vi "eventstructure.vi"() -> ()   [LabVIEW 2017]
uses:
  <vilib>/event_ctls.llb/eventsource.ctl
  <vilib>/event_ctls.llb/lveventtype.ctl
panel:
  out "Time":u32
  out "Type":T1=enum."Value Change"
  out "Source":T2 items=["LabVIEW UI"=0, "ActiveX"=1, "User Event"=25]
  in  "Tab Control":enum32{"Page 1", "Page 2"}(tab)
  in  "Slide":dbl(slide) scale=0.0..10.0
  in  "Slide 2":dbl(slide) scale=0.0..10.0
  out "Knob":dbl(knob) scale=0.0..100.0
  out "Numeric":i32
  in  "stop":bool
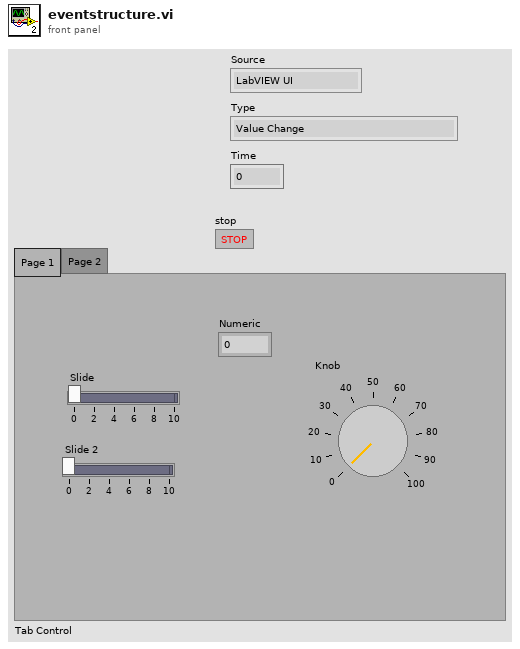
[diagram p1: front panel]
types:
  T1 = typedef "lveventtype.ctl" = enum32{"Null", "Timeout", "Annotation Menu Selection", "Annotation Menu Selection?", "App Instance Close", "App Instance Close?", "Autoscale Range Change", "Bookmark Info Change", "Cell Edit", "Cell Edit?", "Cursor Grab", "Cursor Grab?", "Cursor Menu Selection", "Cursor Menu Selection?", "Cursor Move", "Cursor Release", "Data Change", "Direction Change", "Display State Change", "Drag Ended", "Drag Enter", "Drag Leave", "Drag Over", "Drag Source Update", "Drag Starting", "Drag Starting?", "Drop", "Exec State Change", "Key Down", "Key Down?", "Key Repeat", "Key Repeat?", "Key Up", "Listbox Double Click", "Menu Activation?", "Menu Selection (App)", "Menu Selection? (App)", "Menu Selection (User)", "Mouse Down", "Mouse Down?", "Mouse Enter", "Mouse Leave", "Mouse Move", "Mouse Up", "Mouse Wheel", "NI Security User Change (App)", "Pane Size", "Panel Close", "Panel Close?", "Panel Resize", "Plot Attribute Change", "Scale Range Change", "Shortcut Menu Activation?", "Shortcut Menu Selection (App)", "Shortcut Menu Selection? (App)", "Shortcut Menu Selection (User)", "Tree Double Click", "Tree Drag", "Tree Drag?", "Tree Drop", "Tree Drop?", "Tree Item Close", "Tree Item Close?", "Tree Item Open", "Tree Item Open?", "User Event", "Value Change"}
  T2 = typedef "eventsource.ctl" = u32
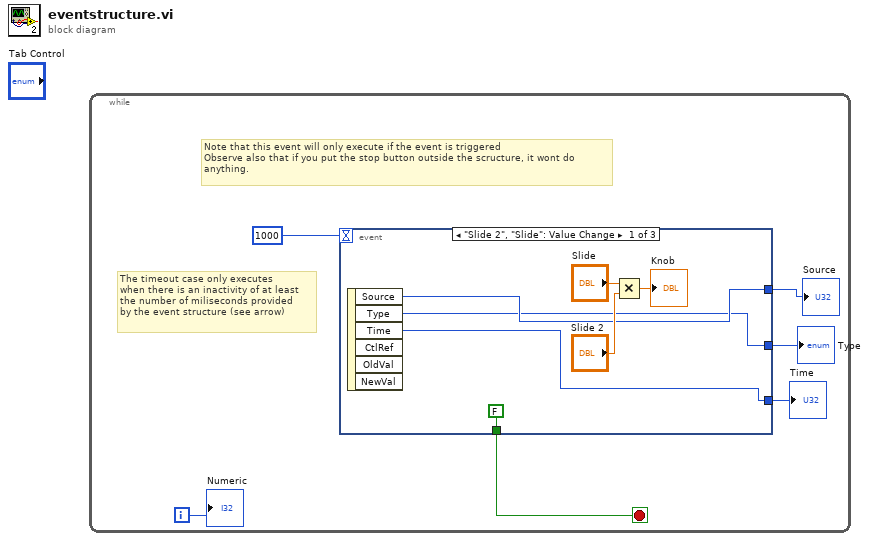
[diagram p0: block diagram]
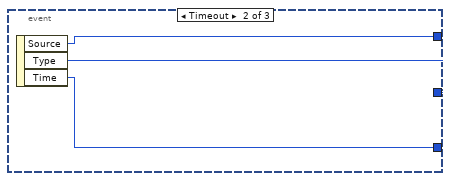
[diagram p2: hidden frame]
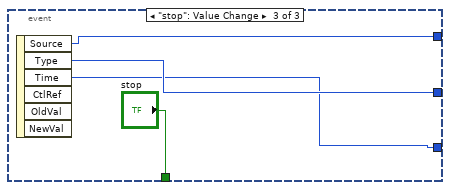
[diagram p3: hidden frame]
diagram:
  n1 = while {
    i -> [w6]
    stop <- w5 stop-if-true
    # "The timeout case only executes\nwhen there is an inactivity of at least\nthe number of miliseconds provided \nby the event structure (see arrow)"
    # "Note that this event will only execute if the event is triggered\nObserve also that if you put the stop button outside the scructure, it wont do \nanything."
    n2 = event shown="[0] \"Slide 2\", \"Slide\": Value Change" {
      selector: _ -> [_ _ _]
      dyn-events: _ -> [_ _ _]
      timeout: 1000 -> [_ _ _]
      tunnel: [FALSE ("stop") _ "stop"] -> w5
      tunnel: [w9 w16 w19] -> w3
      tunnel: [w8 w15 w18] -> w2
      tunnel: [w7 w14 w17] -> w1
      event "Slide 2", "Slide": Value Change {
        n3 = event-data() -> ("Source"=w9:T2, "Type"=w8:T1, "Time"=w7:u32)  [unwired: 1 in, 3 out]
        n4 = Multiply(x="Slide", y="Slide 2") -> (x*y=→"Knob":dbl)
      }
      event Timeout {
        n5 = event-data() -> ("Source"=w16:T2, "Type"=w15:T1, "Time"=w14:u32)  [unwired: 1 in]
      }
      event "stop": Value Change {
        n6 = event-data() -> ("Source"=w19:T2, "Type"=w18:T1, "Time"=w17:u32)  [unwired: 1 in, 3 out]
      }
    }
    "Source" <- w3
    "Type" <- w2
    "Time" <- w1
    "Numeric" <- w6
  }
